vi "make tester present frame.vi"(4 "Cluster::":refnum<k21>, 5 "New Frame Properties":T1={"Comment"="Tester_Present", "Default Payload"=[80], "Identifier"=62, "Name (Short)"="TstrPrsnt", "Payload Length"=1, "PDU_Mapping"=[], "CAN:Extended Identifier?"=FALSE, "CAN:Timing Type"=0, "CAN:Transmit Time"=0.1, "CAN:I/O Mode"=0} {"CAN:I/O Mode" items=["CAN 2.0", "CAN FD", "CAN FD+BRS"]; "Identifier" format="%.0x"; "CAN:Timing Type" items=["Cyclic Data", "Event Data", "Cyclic Remote", "Event Remote", "Cyclic/Event"]; "Default Payload" format="%.0x"}, 6 "frame name":string="Tester_Present", 7 "error in (no error)":errorcluster, 9 "database in":refnum<k21>="MLBevo_KCAN_KMatrix_V8") -> (24 "target cluster out":refnum<k21>, 27 "error out":errorcluster={"status"=TRUE, "code"=-1074384540, "source"="Property Node (arg 6) in make tester present frame.vi \nProperty: PDU_Mapping"})   [LabVIEW 2014]
uses:
  <vilib>/xnet/xnet.llb/XNET Merge Copy Mode.ctl
  <vilib>/xnet/xnet.llb/XNET Database Create (Frame).vi
  <vilib>/xnet/xnet.llb/XNET Database Merge (Cluster).vi
  <resource>/objmgr/xnet.rc
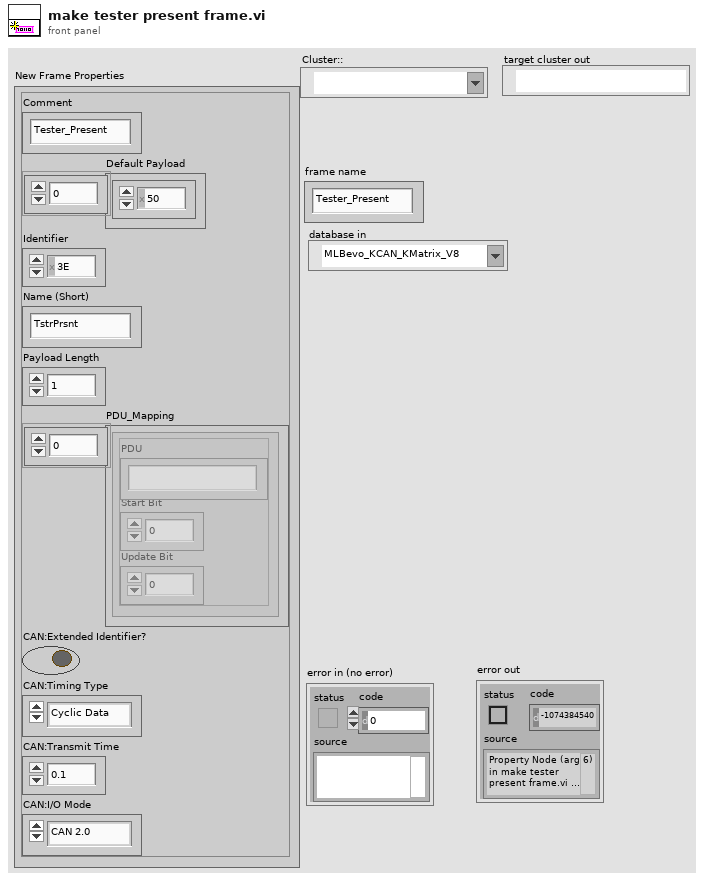
[diagram p1: front panel]
types:
  T1 = cluster{"Comment":string, "Default Payload":u8[], "Identifier":u32, "Name (Short)":string, "Payload Length":u32, "PDU_Mapping":cluster{"PDU":string, "Start Bit":u32, "Update Bit":i32}[], "CAN:Extended Identifier?":bool, "CAN:Timing Type":u32, "CAN:Transmit Time":dbl, "CAN:I/O Mode":u32}
  T2 = typedef "XNET Merge Copy Mode.ctl" = u32
  T3 = cluster{"PDU":string, "Start Bit":u32, "Update Bit":i32}[]
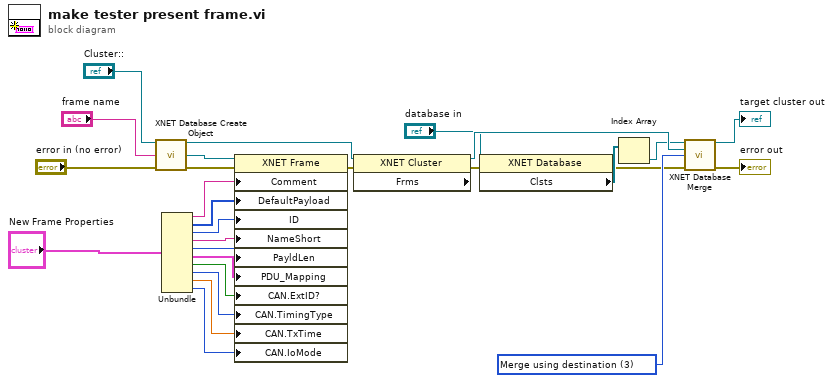
[diagram p0: block diagram]
diagram:
  w24 = T2 3 items=["Copy using source", "Copy using destination", "Merge using source", "Merge using destination"] ("copy mode")
  n1 = call-poly <vilib>:"XNET Database Create Object.vi"("cluster in"="Cluster::", "frame name"="frame name", "error in (no error)"="error in (no error)") -> ("cluster out"=w12:refnum<k21>, "frame out"=w26:refnum<k21>, "error out"=w25:errorcluster)  [unwired: 10 in]
  n2 = Unbundle("New Frame Properties") -> ("Comment"=w22:string, "Default Payload"=w21:u8[], "Identifier"=w20:u32, "Name (Short)"=w19:string, "Payload Length"=w18:u32, "PDU_Mapping"=w17:T3, "CAN:Extended Identifier?"=w16:bool, "CAN:Timing Type"=w15:u32, "CAN:Transmit Time"=w14:dbl, "CAN:I/O Mode"=w13:u32)
  n3 = property class="XNET Frame"(reference=w26, error in=w25, "Comment"=w22, "DefaultPayload"=w21, "ID"=w20, "NameShort"=w19, "PayldLen"=w18, "PDU_Mapping"=w17, "CAN.ExtID?"=w16, "CAN.TimingType"=w15, "CAN.TxTime"=w14, "CAN.IoMode"=w13) -> (error out=w11:errorcluster)  [unwired: 1 out]
  n4 = property class="XNET Cluster" props=["Frms"](reference=w12, error in=w11) -> (reference out=w10:refnum<k21>, error out=w6:errorcluster)  [unwired: 1 out]
  n5 = property class="XNET Database"(reference="database in", error in=w6) -> (error out=w5:errorcluster, "Clsts"=w8:refnum<k21>[])  [unwired: 1 out]
  n6 = Index Array(array=w8) -> (element=w7:refnum<k21>)  [unwired: 1 in]
  n7 = call-poly <vilib>:"XNET Database Merge.vi"("target cluster in"=w7, "source cluster"=w10, "copy mode"=w24, "error in (no error)"=w5) -> ("target cluster out"=→"target cluster out":refnum<k21>, "error out"=→"error out":errorcluster)  [unwired: 9 in, 1 out]
